vi "TurnToAngle.vi"(8 "Error In":errorcluster, 10 "Target Angle":dbl) -> (0 "Error Out":errorcluster)   [LabVIEW 2016]
uses:
  <vilib>/addons/control/pid/pid.llb/PID (DBL).vi
  <vilib>/addons/control/pid/NI_PID_pid.lvlib
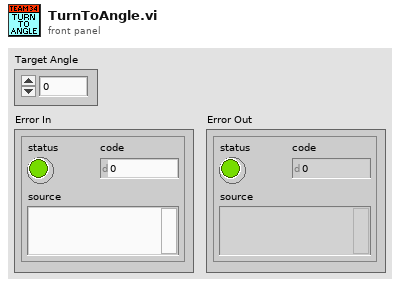
[diagram p1: front panel]
types:
  T1 = typedef "WPI_GyroDevRef.ctl" = cluster{"DevStatus":errorcluster, "Analog Channel":T2, "Offset":dbl, "Gain (VoltsPerDegree/Second)":dbl, "Gyro Type":enum16{"Analog", "XRS450"}, "Handle":i32, "SPI Bus":T3, "Device Found":bool, "Sample Rate":dbl, "Calibrate On Open":bool}
  T2 = typedef "FPGA_AIChannel.ctl" = enum8{"AI 0", "AI 1", "AI 2", "AI 3", "AI MXP 0", "AI MXP 1", "AI MXP 2", "AI MXP 3", "Invalid"}
  T3 = typedef "spi_bus.ctl" = enum16{"SPI On-Board, CS0", "SPI On-Board, CS1", "SPI On-Board, CS2", "SPI On-Board, CS3", "SPI MXP", "Invalid"}
  T4 = cluster{"proportional gain (Kc)":dbl, "integral time (Ti, min)":dbl, "derivative time (Td, min)":dbl}
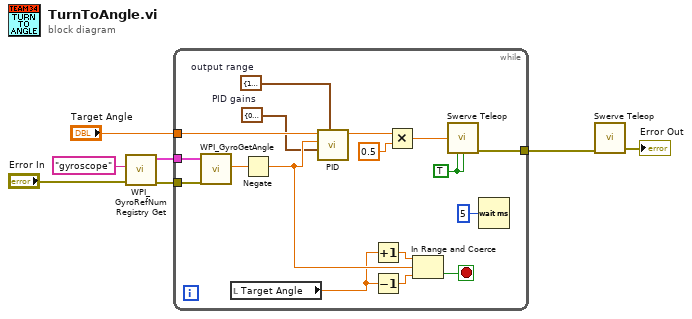
[diagram p0: block diagram]
diagram:
  n1 = call <vilib>:"WPI_GyroRefNum Registry Get.vi"("error in (no error)"="Error In", "refnum name"="gyroscope") -> ("error out"=w7:errorcluster, "GyroDevRef"=w6:T1)  [unwired: 8 in]
  n2 = while {
    tunnel: [w22] -> w4
    tunnel: w6 -> [w16]
    tunnel: w7 -> [w17]
    tunnel: "Target Angle" -> [w11]
    stop <- w18 stop-if-true
    w8 = T4 {"proportional gain (Kc)"=0.04, "integral time (Ti, min)"=0.0, "derivative time (Td, min)"=0.0}  # PID gains
    w9 = cluster{"output high":dbl, "output low":dbl} {"output high"=1.0, "output low"=-1.0}  # output range
    w21 = TRUE ("Robot Centric?")
    n3 = call <vilib>:"WPI_GyroGetAngle.vi"("error in"=w17, "GyroDevRef"=w16) -> ("Angle"=w14:dbl)  [unwired: 5 in, 4 out]
    n4 = local read "Target Angle"() -> (w10:dbl)
    n5 = Negate(x=w14) -> (-x=w13:dbl)
    n6 = call-poly <vilib>:"PID.vi"("output range"=w9, "PID gains"=w8, "process variable"=w13, "setpoint"=w11) -> ("output"=w24:dbl)  [unwired: 6 in, 1 out]
    n7 = Increment(x=w10) -> (x+1=w20:dbl)
    n8 = Decrement(x=w10) -> (x-1=w19:dbl)
    n9 = Multiply(x=w24, y=0.5) -> (x*y=w15:dbl)
    n10 = In Range and Coerce(upper limit=w20, x=w13, lower limit=w19) -> (In Range?=w18:bool)  [unwired: 1 out]
    n11 = call "Swerve Teleop.vi"("Z"=w15, "Robot Centric?"=w21, "Autonomous?"=w21) -> ("Error Out"=w22:errorcluster)  [unwired: 8 in, 4 out]
    n12 = Wait (ms)(milliseconds to wait=u32 5) -> ()  [unwired: 1 out]
  }
  n13 = call "Swerve Teleop.vi"("Error In"=w4) -> ("Error Out"=→"Error Out":errorcluster)  [unwired: 10 in, 4 out]
